vi "Read Power Supply Information.vi"(8 "error in (no error)":errorcluster, 11 "Lotis in":refnum<class "PL Lotis TII LS.lvclass">) -> (0 "error out":errorcluster, 2 "information":T1, 3 "Lotis out":refnum<class "PL Lotis TII LS.lvclass">)   [LabVIEW 2015, in "PL Lotis TII LS.lvclass"]
doc: "Reads power supply information."
uses:
  PL Lotis TII LS.lvclass
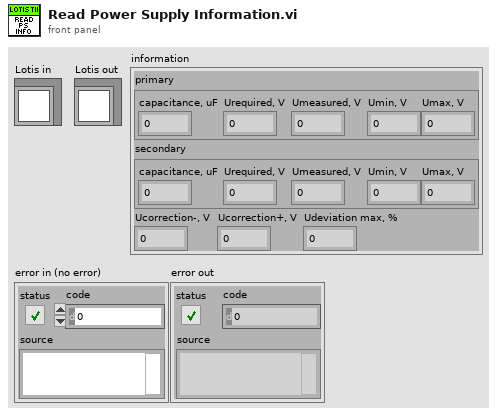
[diagram p1: front panel]
types:
  T1 = cluster{"primary":cluster{"capacitance, uF":u32, "Urequired, V":u32, "Umeasured, V":u32, "Umin, V":u32, "Umax, V":u32}, "secondary":cluster{"capacitance, uF":u32, "Urequired, V":u32, "Umeasured, V":u32, "Umin, V":u32, "Umax, V":u32}, "Ucorrection-, V":u32, "Ucorrection+, V":u32, "Udeviation max, %":u32}
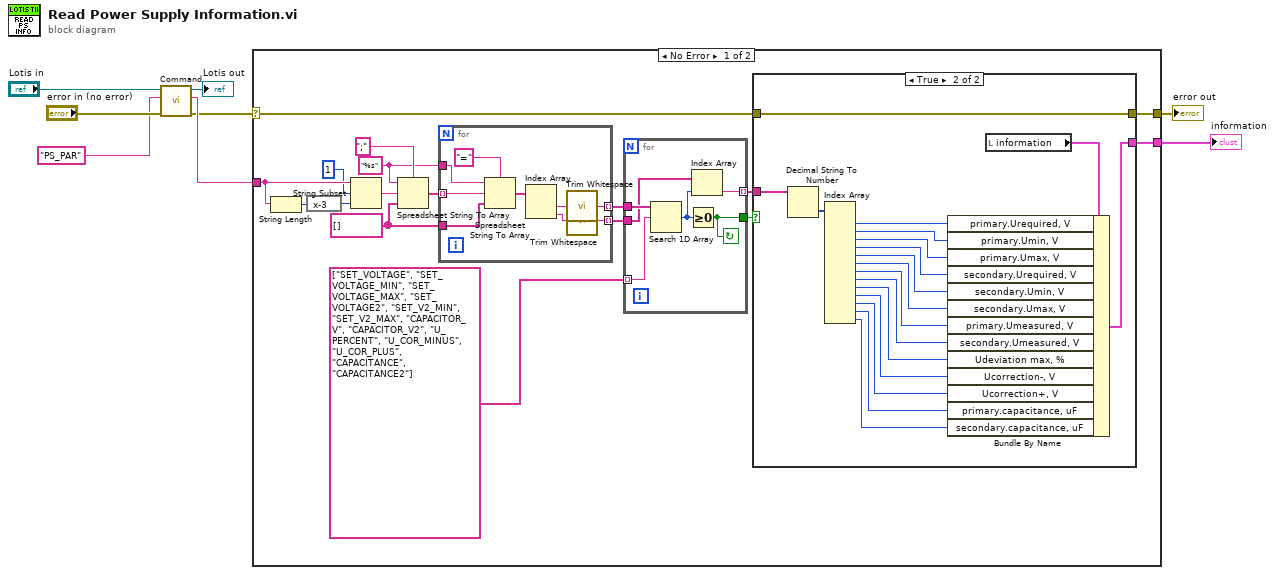
[diagram p0: block diagram]
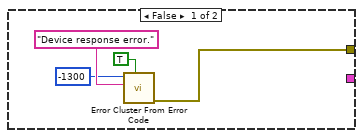
[diagram p2: hidden frame]
diagram:
  n1 = call "Command.vi"("error in (no error)"="error in (no error)", "command"="PS_PAR", "Lotis in"="Lotis in") -> ("error out"=w3:errorcluster, "response data"=w4:string, "Lotis out"=→"Lotis out":refnum<class "PL Lotis TII LS.lvclass">)  [unwired: 6 in]
  n2 = case shown="No Error" w3 {
    selector: w3 -> [w14 w63]
    tunnel: w4 -> [w25 _]
    tunnel: [w13 w63] -> w2
    tunnel: [w9 _] -> w1
    frame No Error {
      w18 = "%s" ("format string")
      w17 = string[] [] ("array type (2D Dbl)")
      n3 = String Length(string=w25) -> (length=w23:i32)
      n4 = expression code="x-3"(w23) -> (w22:i32)
      n5 = String Subset(string=w25, offset (0)=1, length (rest)=w22) -> (substring=w21:string)
      n6 = Spreadsheet String To Array(delimiter (Tab)=";", format string=w18, spreadsheet string=w21, array type (2D Dbl)=w17) -> (array=w19:string[])
      n7 = for {
        tunnel: w19 -> [w59] mode=indexing
        tunnel: w18 -> [w62]
        tunnel: w17 -> [w60]
        tunnel: [w55] -> w16 mode=indexing
        tunnel: [w54] -> w11 mode=indexing
        n8 = Spreadsheet String To Array(delimiter (Tab)="=", format string=w62, spreadsheet string=w59, array type (2D Dbl)=w60) -> (array=w58:string[])
        n9 = Index Array(array=w58) -> (element #1=w57:string, element #2=w56:string)  [unwired: 2 in]
        n10 = call <vilib>:"Trim Whitespace.vi"("string"=w57) -> ("trimmed string"=w55:string)  [unwired: 1 in]
        n11 = call <vilib>:"Trim Whitespace.vi"("string"=w56) -> ("trimmed string"=w54:string)  [unwired: 1 in]
      }
      n12 = for {
        tunnel: w16 -> [w53]
        tunnel: string[] ["SET_VOLTAGE", "SET_VOLTAGE_MIN", "SET_VOLTAGE_MAX", "SET_VOLTAGE2", "SET_V2_MIN", "SET_V2_MAX", "CAPACITOR_V", "CAPACITOR_V2", "U_PERCENT", "U_COR_MINUS", "U_COR_PLUS", "CAPACITANCE", "CAPACITANCE2"] -> [w52] mode=indexing
        tunnel: [w51] -> w12
        tunnel: w11 -> [w50]
        tunnel: [w48] -> w10 mode=indexing
        stop <- w51 continue-if-true
        n13 = Search 1D Array(1D array=w53, element=w52) -> (index of element=w49:i32)  [unwired: 1 in]
        n14 = Greater Or Equal To 0?(x=w49) -> (x >= 0?=w51:bool)
        n15 = Index Array(array=w50, index=w49) -> (element=w48:string)
      }
      n16 = case shown="True" w12 {
        tunnel: w14 -> [_ w47]
        tunnel: [w26 w47] -> w13
        tunnel: w10 -> [_ w44]
        tunnel: [_ w45] -> w9
        frame False {
          n17 = call <vilib>:"Error Cluster From Error Code.vi"("show call chain? (False)"=TRUE, "error message (\"\")"="Device response error." ("format string"), "error code (0)"=-1300) -> ("error out"=w26:errorcluster)  [unwired: 6 in]
        }
        frame True {
          n18 = Decimal String To Number(string=w44) -> (number=w43:i32[])  [unwired: 2 in, 1 out]
          n19 = Index Array(array=w43) -> (element #1=w42:i32, element #2=w41:i32, element #3=w40:i32, element #4=w39:i32, element #5=w38:i32, element #6=w37:i32, element #7=w36:i32, element #8=w35:i32, element #9=w34:i32, element #10=w33:i32, element #11=w32:i32, element #12=w31:i32, element #13=w30:i32)  [unwired: 13 in]
          n20 = local read "information"() -> (w46:T1)
          n21 = Bundle By Name(cluster=w46, "primary.Urequired, V"=w42, "primary.Umin, V"=w41, "primary.Umax, V"=w40, "secondary.Urequired, V"=w39, "secondary.Umin, V"=w38, "secondary.Umax, V"=w37, "primary.Umeasured, V"=w36, "secondary.Umeasured, V"=w35, "Udeviation max, %"=w34, "Ucorrection-, V"=w33, "Ucorrection+, V"=w32, "primary.capacitance, uF"=w31, "secondary.capacitance, uF"=w30) -> (w45:T1)
        }
      }
    }
    frame Error {
    }
  }
  "error out" <- w2
  "information" <- w1
